vi "Tester.vi"() -> ()   [LabVIEW 2020, in "Process Generator.lvclass"]
uses:
  Process Generator.lvclass
  Process Generator.lvclass/Process Generator.ctl
  Framework/Process/Process.lvclass
  Framework Test/Process Test/Process Test.lvclass
  C:/Users/anton/Documents/GitHub/Triarc-Framework/source/Framework Test/Base Class Test/Base Class Test.lvclass
  C:/Program Files (x86)/National Instruments/LabVIEW 2020/vi.lib/Asteme/LUnit/Test Case.lvclass
  C:/Users/anton/Documents/GitHub/Triarc-Framework/source/Framework Test/Process Test/Process Test.lvclass
panel:
  in  "Numeric":i32=15
  out "error out":errorcluster
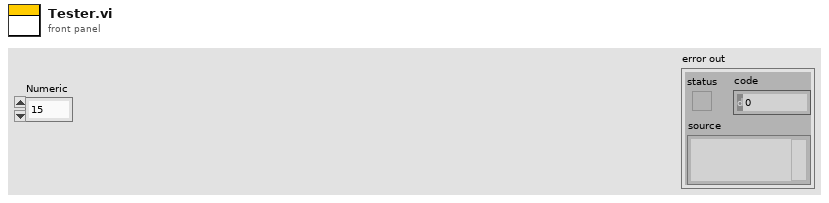
[diagram p1: front panel]
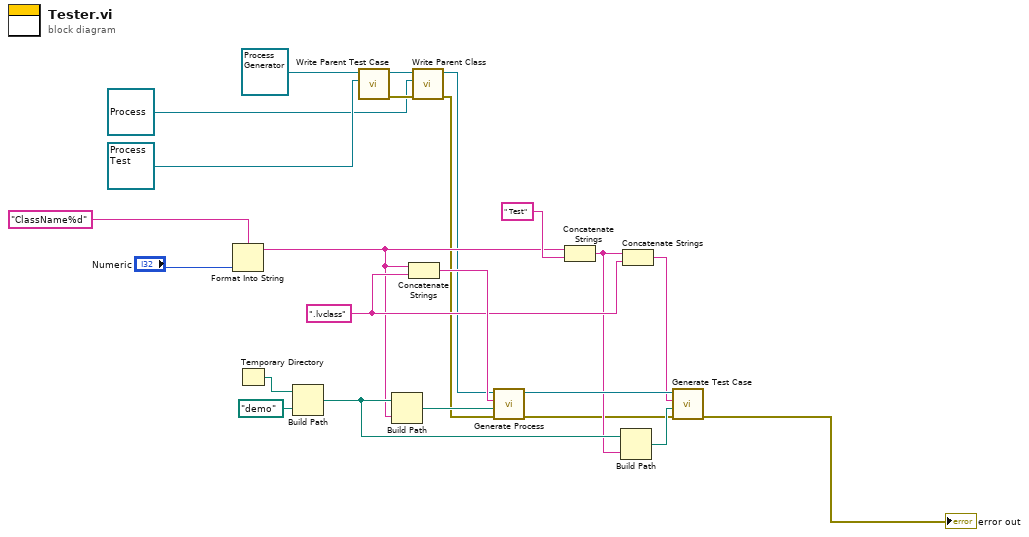
[diagram p0: block diagram]
diagram:
  w15 = ".lvclass" ("string")
  n1 = Format Into String(format string="ClassName%d", "Numeric") -> (resulting string=w10:string)  [unwired: 2 in, 1 out]
  n2 = Temporary Directory() -> (w23:path)
  n3 = Build Path(base path=w23, name or relative path=path "demo") -> (appended path=w17:path)
  n4 = call "Write Parent Test Case.vi"("Parent Test Case"=refnum<class "Process Test.lvclass"> refnum ("Process Test.lvclass"), "Process Generator In"=refnum<class "Process Generator.lvclass"> refnum) -> ("error out"=w5:errorcluster, "Process Generator Out"=w6:refnum<class "Process Generator.lvclass">)  [unwired: 8 in]
  n5 = Build Path(base path=w17, name or relative path=w10) -> (appended path=w21:path)
  n6 = Concatenate Strings(w10, w15) -> (w19:string)
  n7 = call "Write Parent Class.vi"("error in (no error)"=w5, "Parent Process"=refnum<class "Process.lvclass"> refnum ("Parent Class"), "Process Generator In"=w6) -> ("error out"=w4:errorcluster, "Process Generator Out"=w1:refnum<class "Process Generator.lvclass">)  [unwired: 7 in]
  n8 = call "Generate Process.vi"("error in (no error)"=w4, "Directory"=w21, "Name"=w19, "Process Generator In"=w1) -> ("error out"=w12:errorcluster, "Process Generator Out"=w20:refnum<class "Process Generator.lvclass">)  [unwired: 6 in]
  n9 = Concatenate Strings(w10, " Test" ("string")) -> (w14:string)
  n10 = Build Path(base path=w17, name or relative path=w14) -> (appended path=w13:path)
  n11 = Concatenate Strings(w14, w15) -> (w16:string)
  n12 = call "Generate Test Case.vi"("error in (no error)"=w12, "Directory"=w13, "Name"=w16, "Process Generator In"=w20) -> ("error out"=→"error out":errorcluster)  [unwired: 6 in, 1 out]
